vi "Control Switches DAO.vi"(8 "error in (no error)":errorcluster, 10 "Control Loop Switches In":T2, 11 "DAO Actions":T1) -> (0 "error out":errorcluster, 2 "Control Loop Switches Out":T2)   [LabVIEW 2009]
uses:
  Control Loop Switches.ctl
  Control Loop State.ctl
  Apps/On Off Button.ctl
  Data Access Objects/Metadata/DAO Actions.ctl
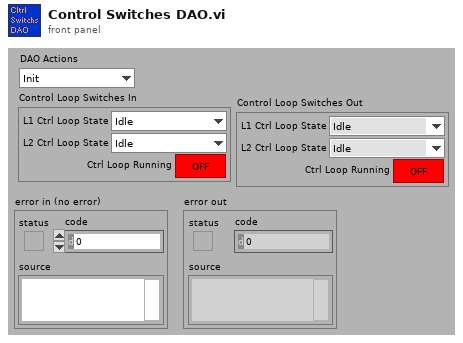
[diagram p1: front panel]
types:
  T1 = typedef "DAO Actions.ctl" = enum16{"Init", "Get", "Set"}
  T2 = typedef "Control Loop Switches.ctl" = cluster{"L1 Ctrl Loop State":T3, "L2 Ctrl Loop State":T3, "Step-wise Data":T4}
  T3 = typedef "Control Loop State.ctl" = enum16{"Idle", "Off", "Reset Autobalancing", "Autobalancing", "Set Command", "Ready for Control", "On"}
  T4 = typedef "On Off Button.ctl" = bool
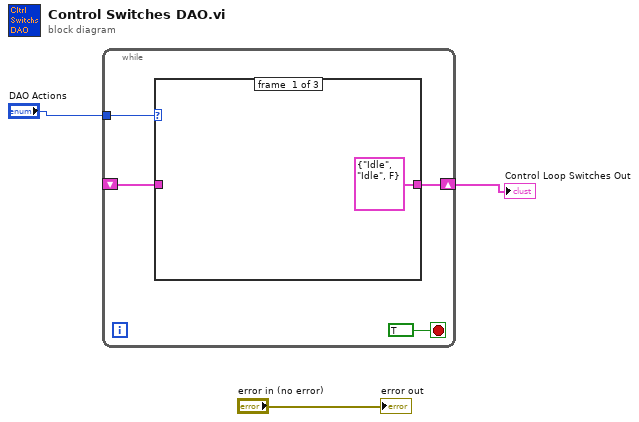
[diagram p0: block diagram]
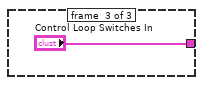
[diagram p3: hidden frame]
diagram:
  n1 = while {
    tunnel: "DAO Actions" -> [w6]
    shift-right: [w5] -> w2
    shift-left: _ -> [w4]
    stop <- TRUE stop-if-true
    n2 = case shown="\"Init\"" w6 {
      tunnel: [T2 {"L1 Ctrl Loop State"=enum."Idle", "L2 Ctrl Loop State"=enum."Idle", "Step-wise Data"=FALSE} ("Control Loop Switches In") w9 "Control Loop Switches In"] -> w5
      tunnel: w4 -> [_ w9 _]
      frame #0 {
      }
      frame #1 {
      }
      frame #2 {
      }
    }
  }
  "Control Loop Switches Out" <- w2
  "error out" <- "error in (no error)"
